vi "Get motor command.vi"(10 "Direction (F = Backward)":bool, 11 "Avance":dbl) -> (3 "Datos Zaber":T1)   [LabVIEW 2020]
uses:
  Type Definitions/Datos Zaber.ctl
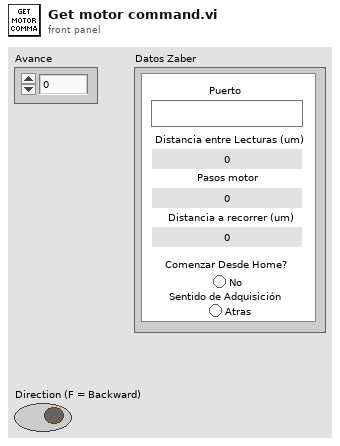
[diagram p1: front panel]
types:
  T1 = typedef "Datos Zaber.ctl" = cluster{"Sentido de Adquisición":bool, "Comenzar Desde Home?":bool, "Distancia a recorrer (um)":dbl, "Pasos motor":i32, "Distancia entre Lecturas (um)":dbl, "Puerto":refnum<visa-resource-name>}
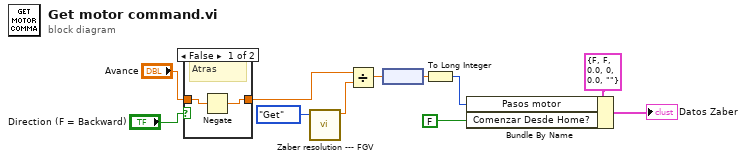
[diagram p0: block diagram]
diagram:
  n1 = case shown="False" "Direction (F = Backward)" {
    tunnel: "Avance" -> [w13 w14]
    tunnel: [w12 w14] -> w7
    frame False {
      # "Atras"
      n2 = Negate(x=w13) -> (-x=w12:dbl)
    }
    frame True {
      # "Adelante"
    }
  }
  n3 = call "Zaber resolution --- FGV.vi"("Action"=enum16{"Get", "Set"}."Get") -> ("Resolución"=w8:dbl[unit])  [unwired: 10 in]
  n4 = Divide(x=w7, y=w8) -> (x/y=w10:dbl[unit])
  n5 = node(w10) -> (w9:dbl)
  n6 = To Long Integer(number=w9) -> (32bit integer=w11:i32)
  n7 = Bundle By Name(cluster=T1 {"Sentido de Adquisición"=FALSE, "Comenzar Desde Home?"=FALSE, "Distancia a recorrer (um)"=0.0, "Pasos motor"=0, "Distancia entre Lecturas (um)"=0.0, "Puerto"=""} ("Datos Zaber"), "Pasos motor"=w11, "Comenzar Desde Home?"=FALSE) -> (→"Datos Zaber":T1)
